vi "read keyword.vi"(8 "error in (no error)":errorcluster, 10 "keyword":string, 11 "Simulated_Header in":refnum<class "Simulated_Header.lvclass">) -> (0 "error out":errorcluster, 2 "value":string, 3 "Simulated_Header out":refnum<class "Simulated_Header.lvclass">)   [LabVIEW 2018, in "Simulated_Header.lvclass"]
uses:
  Simulated_Header.lvclass
  Simulated_Header.lvclass/Simulated_Header.ctl
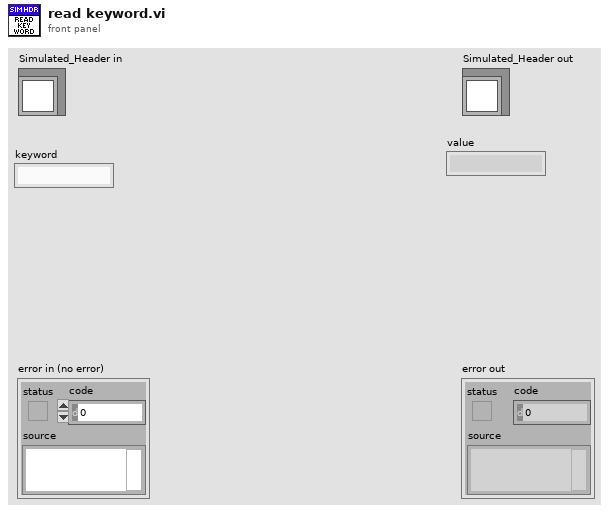
[diagram p1: front panel]
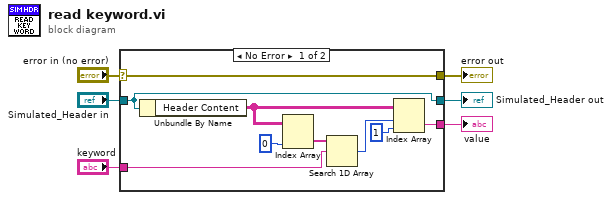
[diagram p0: block diagram]
diagram:
  n1 = case shown="No Error" "error in (no error)" {
    selector: "error in (no error)" -> [w15 w17]
    tunnel: [w15 w17] -> w5
    tunnel: [w14 w16] -> w3
    tunnel: "Simulated_Header in" -> [w14 w16]
    tunnel: "keyword" -> [w11 _]
    tunnel: [w7 _] -> w1
    frame No Error {
      n2 = Unbundle By Name(w14) -> ("Header Content"=w10:string[][])
      n3 = Index Array(array=w10, index (col)=0 ("disabled index (col)")) -> (element=w13:string[])  [unwired: 1 in]
      n4 = Search 1D Array(1D array=w13, element=w11) -> (index of element=w9:i32)  [unwired: 1 in]
      n5 = Index Array(array=w10, index (row)=w9, index (col)=1 ("disabled index (col)")) -> (element=w7:string)
    }
    frame Error {
    }
  }
  "error out" <- w5
  "Simulated_Header out" <- w3
  "value" <- w1
